vi "RequestsJasonToRequestObjectArray.vi"(8 "error in (no error)":errorcluster, 11 "Requests":string) -> (0 "error out":errorcluster, 3 "REquests":refnum<class "Request.lvclass">[](array[class]))   [LabVIEW 2015]
uses:
  LVClasses/Request/Request.lvclass
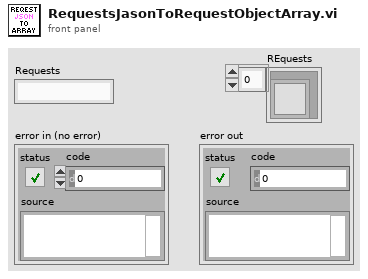
[diagram p1: front panel]
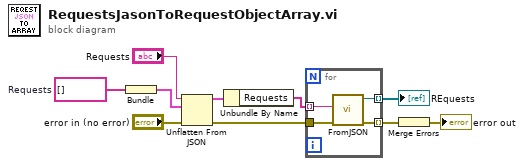
[diagram p0: block diagram]
diagram:
  w8 = string[] []  # Requests
  n1 = Bundle("Requests"=w8) -> (w7:cluster{"Requests":string[]})  [unwired: 1 in]
  n2 = Unflatten From JSON(JSON string="Requests", type and defaults=w7, error in (no error)="error in (no error)") -> (value=w6:cluster{"Requests":string[]}, error out=w1:errorcluster)  [unwired: 4 in]
  n3 = Unbundle By Name(w6) -> ("Requests"=w5:string[])
  n4 = for {
    tunnel: w5 -> [w14] mode=indexing
    tunnel: [w13] -> w4 mode=indexing
    tunnel: [w12] -> w3 mode=indexing
    tunnel: w1 -> [w11]
    n5 = call "FromJSON.vi"("error in (no error)"=w11, "Request"=w14) -> ("error out"=w12:errorcluster, "Request out"=w13:refnum<class "Request.lvclass">)  [unwired: 8 in]
  }
  "REquests" <- w4
  n6 = Merge Errors(w3) -> (→"error out":errorcluster)
